vi "Set Visibility.vi"(8 "error in (no error)":errorcluster, 9 "Visible? (F)":bool, 10 "Channel in":i32, 11 "Graph Manager in":refnum<class "Graph Manager.lvclass">) -> (0 "error out":errorcluster, 2 "Channel out":i32, 3 "Graph Manager out":refnum<class "Graph Manager.lvclass">)   [LabVIEW 2016, in "Graph Manager.lvclass"]
uses:
  Graph Manager.lvclass
  Graph Manager.lvclass/Graph Manager.ctl
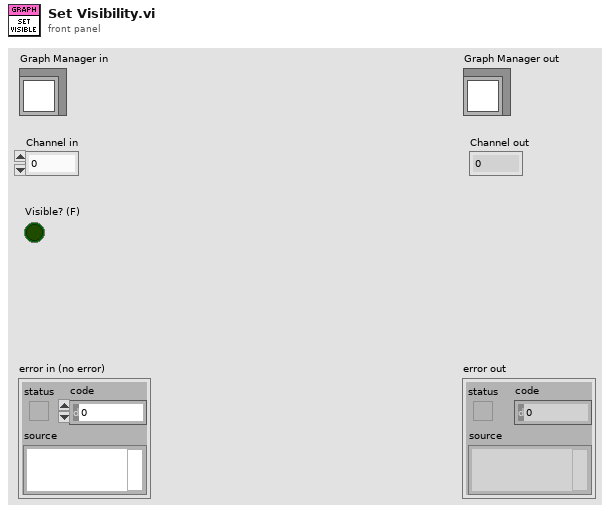
[diagram p1: front panel]
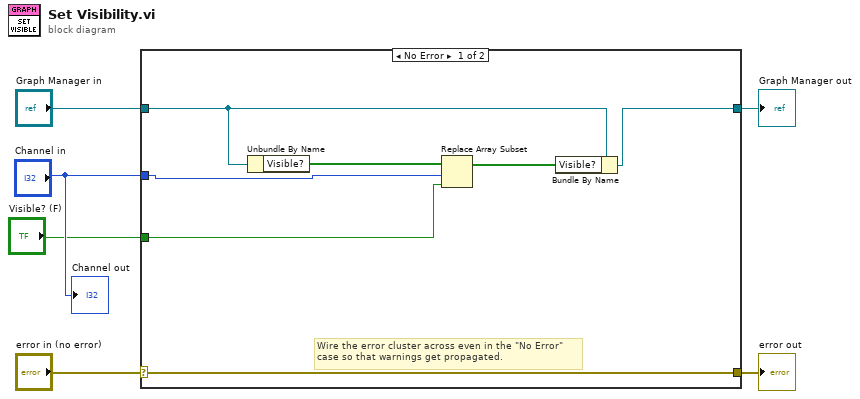
[diagram p0: block diagram]
diagram:
  n1 = case shown="No Error" "error in (no error)" {
    selector: "error in (no error)" -> [w13 w15]
    tunnel: [w13 w15] -> w5
    tunnel: [w9 w14] -> w3
    tunnel: "Graph Manager in" -> [w10 w14]
    tunnel: "Channel in" -> [w7 _]
    tunnel: "Visible? (F)" -> [w11 _]
    frame No Error {
      # "Wire the error cluster across even in the \"No Error\"\ncase so that warnings get propagated."
      n2 = Unbundle By Name(w10) -> ("Visible?"=w12:bool[])
      n3 = Replace Array Subset(array=w12, new element=w11, index=w7) -> (w8:bool[])
      n4 = Bundle By Name(cluster=w10, "Visible?"=w8) -> (w9:refnum<class "Graph Manager.lvclass">)
    }
    frame Error {
    }
  }
  "error out" <- w5
  "Graph Manager out" <- w3
  "Channel out" <- "Channel in"
